vi "Simple RT Add-teardown.vi"(7 "test case ID":string, 10 "Actual x + y result":dbl) -> (3 "result":bool)   [LabVIEW 2018]
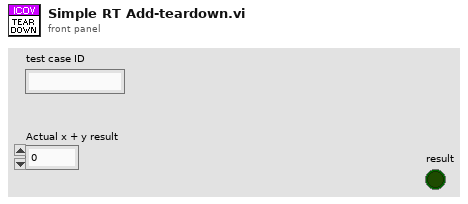
[diagram p1: front panel]
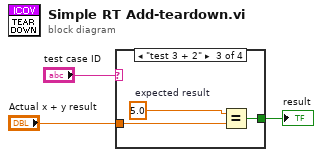
[diagram p0: block diagram]
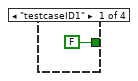
[diagram p2: hidden frame]
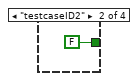
[diagram p3: hidden frame]
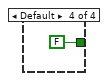
[diagram p4: hidden frame]
diagram:
  n1 = case shown="\"test 3 + 2\"" "test case ID" {
    tunnel: [FALSE FALSE w6 FALSE] -> w2
    tunnel: "Actual x + y result" -> [_ _ w7 _]
    frame "testcaseID1" {
    }
    frame "testcaseID2" {
    }
    frame "test 3 + 2" {
      w8 = 5.0  # expected result
      n2 = Equal?(x=w8, y=w7) -> (x = y?=w6:bool)
    }
    frame Default {
    }
  }
  "result" <- w2
